vi "Set Frequency Data.vi"(8 "error in (no error)":errorcluster, 11 "Skyworks Spur Test in":refnum<class "Skyworks Spur Test.lvclass">) -> (0 "error out":errorcluster, 3 "Skyworks Spur Test out":refnum<class "Skyworks Spur Test.lvclass">)   [LabVIEW 2018, in "Skyworks Spur Test.lvlib" / "Skyworks Spur Test.lvclass"]
uses:
  Skyworks Spur Test.lvclass
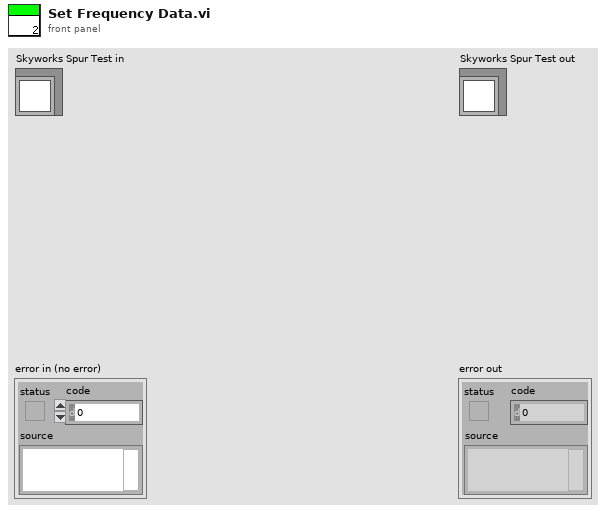
[diagram p1: front panel]
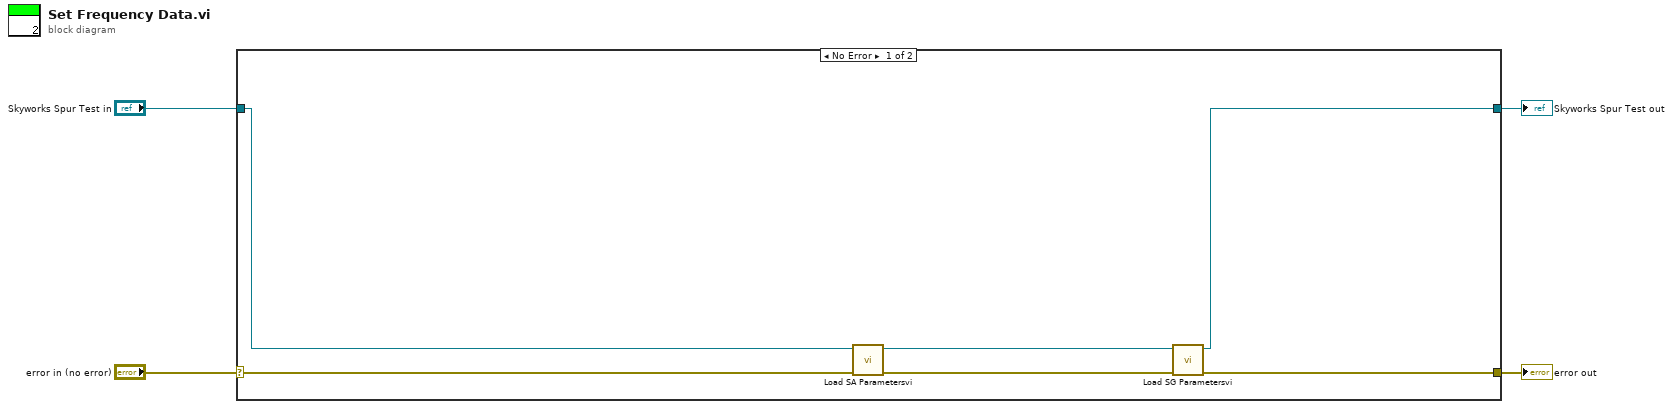
[diagram p0: block diagram]
diagram:
  n1 = case shown="No Error" "error in (no error)" {
    selector: "error in (no error)" -> [w10 w12]
    tunnel: [w7 w12] -> w3
    tunnel: [w5 w11] -> w1
    tunnel: "Skyworks Spur Test in" -> [w8 w11]
    frame No Error {
      n2 = call "Load SA Parametersvi.vi"("error in (no error)"=w10, "Skyworks Spur Test in"=w8) -> ("error out"=w9:errorcluster, "Skyworks Spur Test out"=w6:refnum<class "Skyworks Spur Test.lvclass">)  [unwired: 8 in]
      n3 = call "Load SG Parametersvi.vi"("error in (no error)"=w9, "Skyworks Spur Test in"=w6) -> ("error out"=w7:errorcluster, "Skyworks Spur Test out"=w5:refnum<class "Skyworks Spur Test.lvclass">)  [unwired: 8 in]
    }
    frame Error {
    }
  }
  "error out" <- w3
  "Skyworks Spur Test out" <- w1
